vi "TW Resolve gRPC Server Dependencies.vi"(8 "error in":errorcluster, 9 "New Subname":string, 10 "Template Project Path":path, 11 "Map - LibRef":map{string, refnum<vi>}(c390)) -> (0 "error out":errorcluster)   [LabVIEW 2021, in "Plugin Generator.lvlib"]
uses:
  Plugin Generator.lvlib
  <vilib>/CIF Foundation/CIF LabVIEW Scripting/LV Scripting/LV Scripting Utilities.lvlib
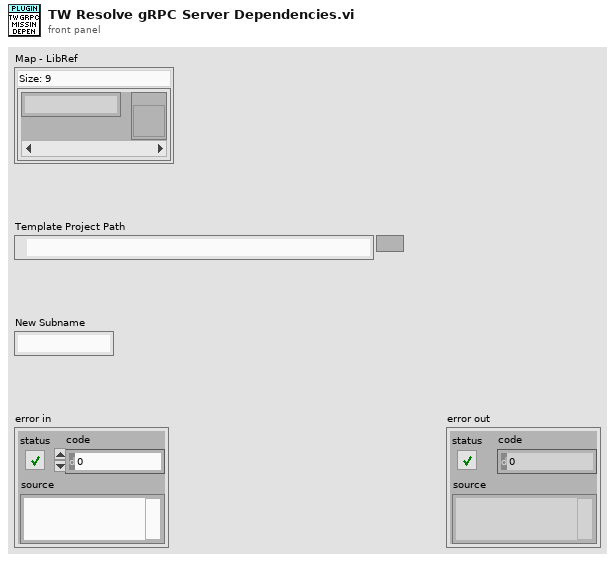
[diagram p1: front panel]
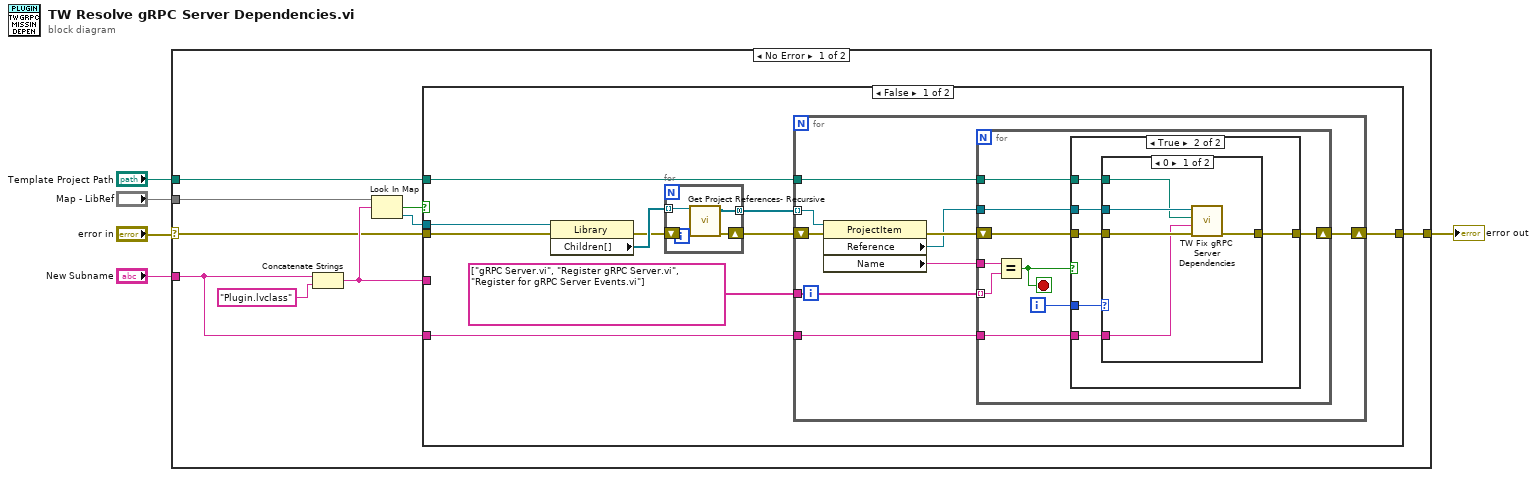
[diagram p0: block diagram]
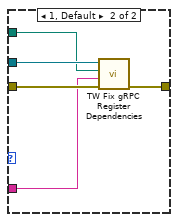
[diagram p3: hidden frame]
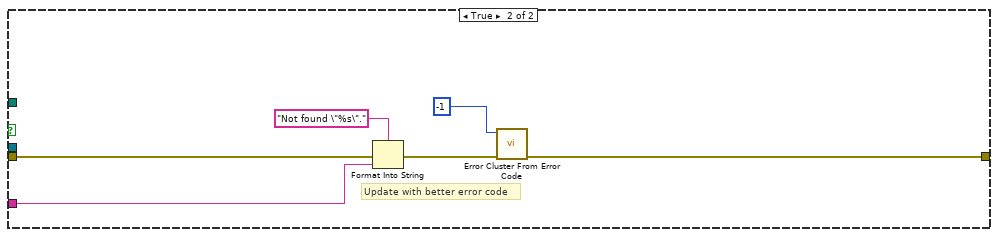
[diagram p4: hidden frame]
diagram:
  n1 = case shown="No Error" "error in" {
    selector: "error in" -> [w6 w70]
    tunnel: [w14 w70] -> w5
    tunnel: "Map - LibRef" -> [w10 _]
    tunnel: "New Subname" -> [w8 _]
    tunnel: "Template Project Path" -> [w7 _]
    frame No Error {
      n2 = Concatenate Strings(w8, "Plugin.lvclass" ("String")) -> (w9:string)
      n3 = Look In Map(map=w10, key=w9) -> (key not found?=w12:bool, value=w13:refnum<vi>)  [unwired: 1 in]
      n4 = case shown="False" w12 {
        tunnel: w13 -> [w24 _]
        tunnel: [w18 w66] -> w14
        tunnel: w8 -> [w19 _]
        tunnel: w9 -> [_ w65]
        tunnel: w7 -> [w17 _]
        tunnel: w6 -> [w15 w64]
        frame False {
          n5 = property class="Library"(reference=w24, error in=w15) -> (error out=w22:errorcluster, "Children[]"=w23:refnum<vi>[])  [unwired: 1 out]
          n6 = for {
            tunnel: w23 -> [w63] mode=indexing
            tunnel: [w62] -> w21 mode=concatenating
            shift-right: [w60] -> w16
            shift-left: w22 -> [w61]
            n7 = call <vilib>:"Get Project References- Recursive.vi"("error in"=w61, "TargetItem in"=w63) -> ("error out"=w60:errorcluster, "TargetItem out"=w62:refnum<vi>[])  [unwired: 8 in]
          }
          n8 = for {
            tunnel: w21 -> [w33] mode=indexing
            tunnel: string[] ["gRPC Server.vi", "Register gRPC Server.vi", "Register for gRPC Server Events.vi"] -> [w32]
            tunnel: w17 -> [w28]
            tunnel: w19 -> [w27]
            shift-right: [w26] -> w18
            shift-left: w16 -> [w31]
            n9 = property class="ProjectItem"(reference=w33, error in=w31) -> (error out=w30:errorcluster, "Reference"=w29:refnum<vi>, "Name"=w25:string)  [unwired: 1 out]
            n10 = for {
              tunnel: w32 -> [w42] mode=indexing
              tunnel: w25 -> [w41]
              tunnel: w29 -> [w39]
              tunnel: w28 -> [w36]
              tunnel: w27 -> [w35]
              shift-right: [w34] -> w26
              shift-left: w30 -> [w40]
              i -> [w37]
              stop <- w38 stop-if-true
              n11 = Equal?(x=w41, y=w42) -> (x = y?=w38:bool)
              n12 = case shown="True" w38 {
                tunnel: w40 -> [w43 w48]
                tunnel: w39 -> [_ w49]
                tunnel: w37 -> [_ w47]
                tunnel: w36 -> [_ w46]
                tunnel: w35 -> [_ w45]
                tunnel: [w43 w44] -> w34
                frame False {
                }
                frame True {
                  n13 = case shown="0" w47 {
                    tunnel: w49 -> [w54 w58]
                    tunnel: w48 -> [w53 w59]
                    tunnel: w46 -> [w52 w56]
                    tunnel: w45 -> [w51 w55]
                    tunnel: [w50 w57] -> w44
                    frame 0 {
                      n14 = call "TW Fix gRPC Server Dependencies.vi"("error in"=w53, "gRPC Service Name"=w51, "Project Path"=w52, "VI Refnum"=w54) -> ("error out"=w50:errorcluster)  [unwired: 7 in]
                    }
                    frame 1, Default {
                      n15 = call "TW Fix gRPC Register Dependencies.vi"("error in"=w59, "gRPC Service Name"=w55, "Project Path"=w56, "VI Refnum"=w58) -> ("error out"=w57:errorcluster)  [unwired: 7 in]
                    }
                  }
                }
              }
            }
          }
        }
        frame True {
          # "Update with better error code"
          n16 = Format Into String(format string="Not found \"%s\"." ("error message (\"\")"), error in=w64, w65) -> (error out=w68:errorcluster)  [unwired: 1 in, 1 out]
          n17 = call <vilib>:"Error Cluster From Error Code.vi"("error in (no error)"=w68, "error code (0)"=-1) -> ("error out"=w66:errorcluster)  [unwired: 7 in]
        }
      }
    }
    frame Error {
    }
  }
  "error out" <- w5
